vi "Untitled 2 (SubVI).vi"(8 "error in (no error)":errorcluster, 11 "LINX Resource in":T1) -> (0 "error out":errorcluster, 2 "LINX Resource":T1, 3 "Numeric":dbl)   [LabVIEW 2015]
uses:
  <vilib>/MakerHub/LINX/Private/Type Defs/LINX Ref.ctl
  <vilib>/MakerHub/LINX/Private/Type Defs/Platform.ctl
  <vilib>/MakerHub/LINX/Private/Type Defs/Interface.ctl
  <vilib>/MakerHub/LINX/Private/Device/Type Defs/LINX Device Config.ctl
  <vilib>/MakerHub/LINX/Private/Device/Type Defs/TCP Config.ctl
  <vilib>/MakerHub/LINX/Private/Device/Type Defs/Channels.ctl
  <vilib>/MakerHub/LINX/Private/Local IO/LinxI2cWrite.vi
  <vilib>/MakerHub/LINX/Public/Utilities/Check Channel.vi
  <vilib>/MakerHub/LINX/Private/Utilties/Generate Error.vi
  <vilib>/MakerHub/LINX/LMH-LINX.lvlib
  <vilib>/MakerHub/LINX/Private/Device/Device.lvlib
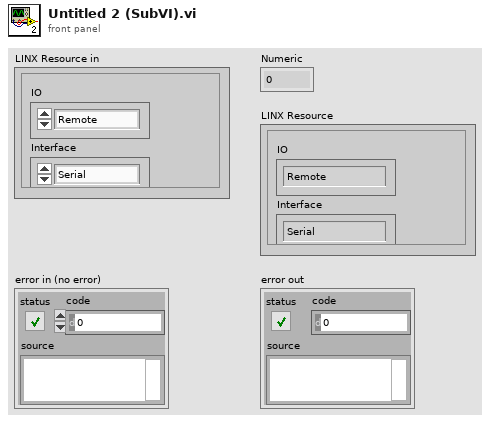
[diagram p1: front panel]
types:
  T1 = typedef "LMH-LINX.lvlib/LINX Ref.ctl" = cluster{"IO":T2, "Interface":T3, "LINX Device Config":T4}
  T2 = typedef "LMH-LINX.lvlib/Platform.ctl" = enum16{"Remote", "Local"}
  T3 = typedef "LMH-LINX.lvlib/Interface.ctl" = enum16{"Serial", "TCP"}
  T4 = typedef "LMH-LINX.lvlib/Device.lvlib/LINX Device Config.ctl" = cluster{"Interface":T3, "COM Port":refnum<visa-resource-name>, "TCP Configuration":T5, "Device Family":u8, "Device ID":u8, "Device Name":string, "TCP Ref":refnum<k5>, "Channels":T6}
  T5 = typedef "LMH-LINX.lvlib/Device.lvlib/TCP Config.ctl" = cluster{"IP Address":string, "Port":u16}
  T6 = typedef "LMH-LINX.lvlib/Channels.ctl" = cluster{"DI":u8[], "DO":u8[], "AI":u8[], "AO":u8[], "PWM":u8[], "QE":u8[], "UART":u8[], "I2C 2":u8[], "SPI":u8[], "CAN":u8[], "Servo":u8[], "AI Ref (V)":dbl, "AI Resolution (Bits)":u8, "AO Ref (V)":dbl, "AO Resolution (Bits)":u8}
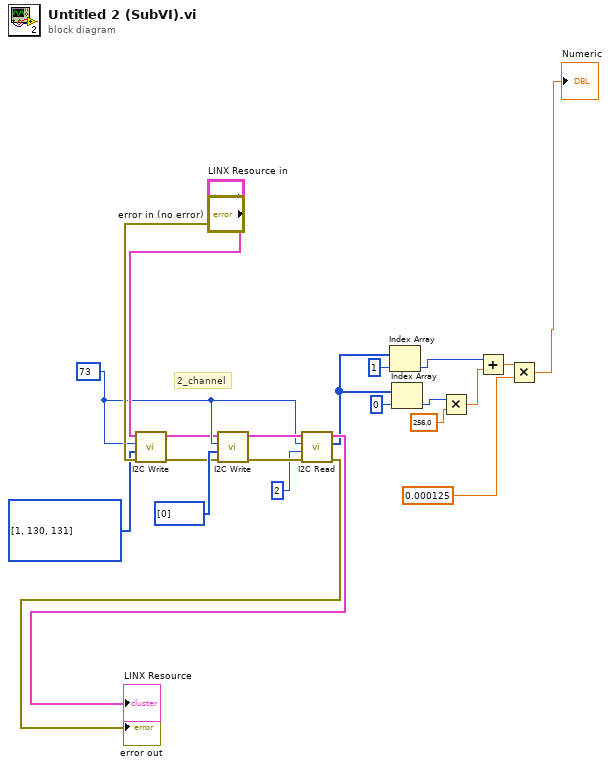
[diagram p0: block diagram]
diagram:
  w3 = 73 ("I2C Slave Address 2")
  # "2_channel"
  n1 = call <vilib>:"I2C Write.vi"("Error In"="error in (no error)", "Data"=u8[] [1, 130, 131], "I2C Slave Address (0)"=w3, "LINX Resource"="LINX Resource in") -> ("Error Out"=w2:errorcluster, "LINX Resource"=w1:T1)  [unwired: 6 in]
  n2 = call <vilib>:"I2C Write.vi"("Error In"=w2, "Data"=u8[] [0], "I2C Slave Address (0)"=w3, "LINX Resource"=w1) -> ("Error Out"=w6:errorcluster, "LINX Resource"=w7:T1)  [unwired: 6 in]
  n3 = call <vilib>:"I2C Read.vi"("Error In"=w6, "Bytes To Read"=u8 2, "I2C Slave Address (0)"=w3, "LINX Resource"=w7) -> ("Error Out"=→"error out":errorcluster, "Data"=w9:u8[], "LINX Resource"=→"LINX Resource":T1)  [unwired: 5 in]
  n4 = Index Array(array=w9, index=1) -> (element=w13:u8)
  n5 = Index Array(array=w9, index=0) -> (element=w12:u8)
  n6 = Multiply(x=w12, y=256.0) -> (x*y=w14:dbl)
  n7 = Add(x=w13, y=w14) -> (x+y=w16:dbl)
  n8 = Multiply(x=w16, y=0.000125) -> (x*y=→"Numeric":dbl)
